vi "Unconstrained Optimization.vi"   [LabVIEW 2017, in "NI_Gmath.lvlib"]
doc: "Solves the unconstrained minimization problem for an arbitrary nonlinear function. You must manually select the polymorphic instance to use."
uses:
  <vilib>/gmath/NI_Gmath.lvlib
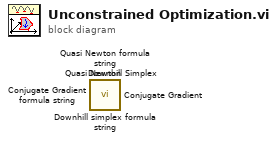
[diagram p0: block diagram]
diagram:
  n1 = call <vilib>:"Downhill simplex formula string.vi"() -> ()  [unwired: 8 in, 4 out]
  n2 = call <vilib>:"Downhill Simplex.vi"() -> ()  [unwired: 8 in, 4 out]
  n3 = call <vilib>:"Conjugate Gradient formula string.vi"() -> ()  [unwired: 8 in, 4 out]
  n4 = call <vilib>:"Conjugate Gradient.vi"() -> ()  [unwired: 8 in, 4 out]
  n5 = call <vilib>:"Quasi Newton formula string.vi"() -> ()  [unwired: 8 in, 4 out]
  n6 = call <vilib>:"Quasi Newton.vi"() -> ()  [unwired: 8 in, 4 out]
